vi "Abort Download.vi"(8 "error in (no error)":errorcluster, 11 "HttpDownloadTask in":T1) -> (0 "error out":errorcluster, 3 "HttpDownloadTask out":T1)   [LabVIEW 2018, in "LabVIEWHTTPClient_NET.lvlib" / "HttpDownloadTask.lvclass"]
uses:
  HttpDownloadTask.lvclass
  Types/DownloadTask_ref.ctl
  HttpDownloadTask.lvclass/HttpDownloadTask.ctl
  Accessors/Read HttpContent out.vi
  HttpContent/HttpContent.lvclass
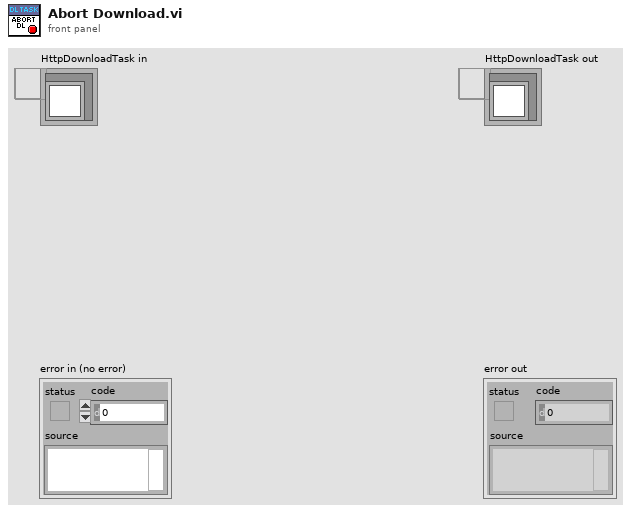
[diagram p1: front panel]
types:
  T1 = typedef "LabVIEWHTTPClient_NET.lvlib/HttpDownloadTask.lvclass/DownloadTask_ref.ctl" = refnum<data-value>
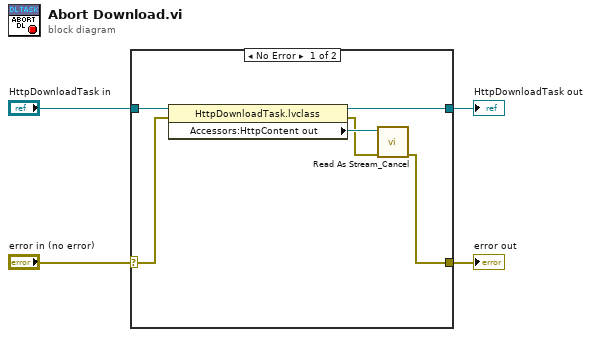
[diagram p0: block diagram]
diagram:
  n1 = case shown="No Error" "error in (no error)" {
    selector: "error in (no error)" -> [w10 w12]
    tunnel: [w5 w12] -> w3
    tunnel: [w8 w11] -> w1
    tunnel: "HttpDownloadTask in" -> [w9 w11]
    frame No Error {
      n2 = property class="HttpDownloadTask.lvclass"(reference=w9, error in=w10) -> (reference out=w8:T1, error out=w6:errorcluster, "Accessors:HttpContent out"=w7:refnum<class "HttpContent.lvclass">)
      n3 = call "Read As Stream_Cancel.vi"("error in (no error)"=w6, "HttpContent in"=w7) -> ("error out"=w5:errorcluster)  [unwired: 8 in, 1 out]
    }
    frame Error {
    }
  }
  "error out" <- w3
  "HttpDownloadTask out" <- w1
